vi "DSF.Shared.Configuration.Transfer.Channel Descriptors Equal.vi"(1 "Channel Descriptor 2":T1 {"VS Channel Ref" format="%016x"; "Channel Parameters"."offset" format="%d bytes"}, 2 "Channel Descriptor 1":T1 {"VS Channel Ref" format="%016x"; "Channel Parameters"."offset" format="%d bytes"}) -> (0 "equal?":bool)   [LabVIEW 2017, in "DSF.Shared.lvlib" / "DSF.Shared.Configuration.Transfer.lvclass"]
uses:
  DSF.Shared.Configuration.Transfer.lvclass
  Typedefs/DSF.Shared.Typedefs.Configuration.Transfer.Channel Descriptor.ctl
  Typedefs/DSF.Shared.Typedefs.Configuration.Transfer.Channel Parameters.ctl
  Typedefs/DSF.Shared.Typedefs.Data Type.ctl
  <vilib>/NI Veristand/Custom Device API/Custom Device Item Ref.ctl
  DSF.Shared.lvlib
  <vilib>/NI Veristand/Custom Device API/Custom Device API.lvlib
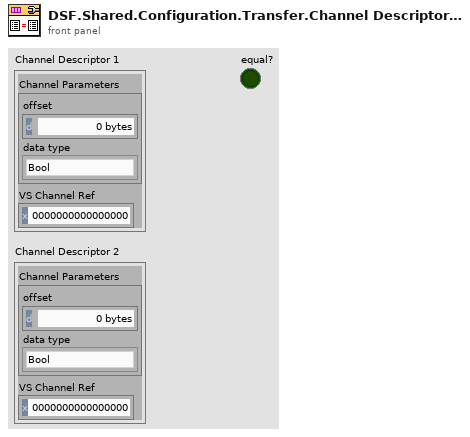
[diagram p1: front panel]
types:
  T1 = typedef "DSF.Shared.lvlib/DSF.Shared.Typedefs.Configuration.Transfer.Channel Descriptor.ctl" = cluster{"Channel Parameters":T2, "VS Channel Ref":T4}
  T2 = typedef "DSF.Shared.lvlib/DSF.Shared.Typedefs.Configuration.Transfer.Channel Parameters.ctl" = cluster{"offset":u64, "data type":T3}
  T3 = typedef "DSF.Shared.lvlib/DSF.Shared.Typedefs.Data Type.ctl" = enum8{"Bool", "SGL", "DBL", "I8", "I16", "I32", "I64", "U8", "U16", "U32", "U64"}
  T4 = typedef "Custom Device API.lvlib/Custom Device Item Ref.ctl" = u64
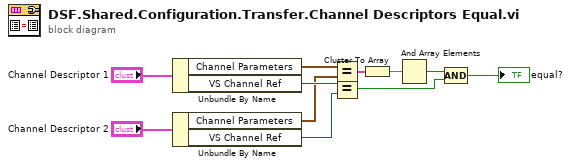
[diagram p0: block diagram]
diagram:
  n1 = Unbundle By Name("Channel Descriptor 1") -> ("Channel Parameters"=w11:T2, "VS Channel Ref"=w10:T4)
  n2 = Unbundle By Name("Channel Descriptor 2") -> ("Channel Parameters"=w8:T2, "VS Channel Ref"=w7:T4)
  n3 = Equal?(x=w11, y=w8) -> (x = y?=w5:cluster{"offset":bool, "data type":bool})
  n4 = Equal?(x=w10, y=w7) -> (x = y?=w6:bool)
  n5 = Cluster To Array(cluster=w5) -> (array=w4:bool[])
  n6 = And Array Elements(Boolean array=w4) -> (logical AND=w3:bool)
  n7 = Compound Arithmetic op=AND(w3, w6) -> (→"equal?":bool)
